vi "fgt get Ttl Channel Count.vi"(8 "error in (no error)":errorcluster) -> (0 "error out":errorcluster, 3 "nbTtlChan out":u32)   [LabVIEW 2016, in "fgt_SDK.lvlib"]
doc: "Get total number of initialized TTL channels. It is the sum of all connected Link TTL ports"
uses:
  fgt_SDK.lvlib
  dlls/fgt_SDK_32.dll
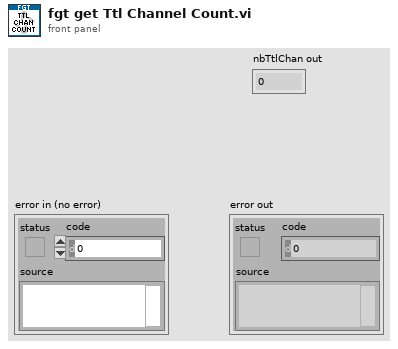
[diagram p1: front panel]
types:
  T1 = typedef "fgt_SDK.lvlib/fgt_STATUS_INFO.ctl" = cluster{"InstrType":T2, "instrSN":u16, "errorCode":u8, "infoCode":u8, "detail":string}
  T2 = typedef "fgt_SDK.lvlib/fgt_INSTRUMENT_TYPE.ctl" = enum32{"None", "MFCS", "MFCS_EZ", "FRP", "LineUP", "IPS"}
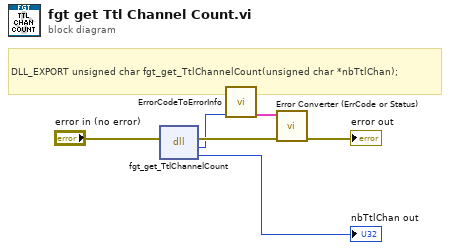
[diagram p0: block diagram]
diagram:
  # "DLL_EXPORT unsigned char fgt_get_TtlChannelCount(unsigned char *nbTtlChan);"
  n1 = dll-call lib="C:/projects/SDK/fgt-sdk-labview/dlls/fgt_SDK_*.*" fn="fgt_get_TtlChannelCount"(error in="error in (no error)") -> (error out=w5:errorcluster, "return type"=w3:u8, "nbTtlChan"=→"nbTtlChan out":u8)  [unwired: 3 in, 1 out]
  n2 = call "ErrorCodeToErrorInfo.vi"("return type"=w3) -> ("StatusInfo"=w2:T1)  [unwired: 10 in]
  n3 = call "Error Converter (ErrCode or Status).vi"("error in (no error)"=w5, "StatusInfo"=w2) -> ("error out"=→"error out":errorcluster)  [unwired: 9 in]
